vi "Pre Launch Init.vi"(11 "Nested in":refnum<class "Save tdms.lvclass">) -> (0 "error out":errorcluster, 3 "Nested out":refnum<class "Save tdms.lvclass">)   [LabVIEW 2019, in "Save tdms.lvlib" / "Save tdms.lvclass"]
doc: "(<B>Filename</B>: Actor Framework.lvlib:Actor.lvclass:Pre Launch Init.vi)\n\nDefines behavior that occurs after the Launch Nested Actor method is invoked but before the actor's Actor Core method begins running.\n\nBy default, this method does nothing. A descendant class may override it to define behavior."
uses:
  Save tdms.lvclass
  <vilib>/ActorFramework/Actor/Actor.lvclass
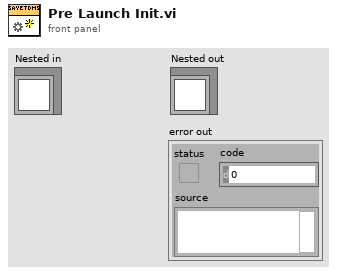
[diagram p1: front panel]
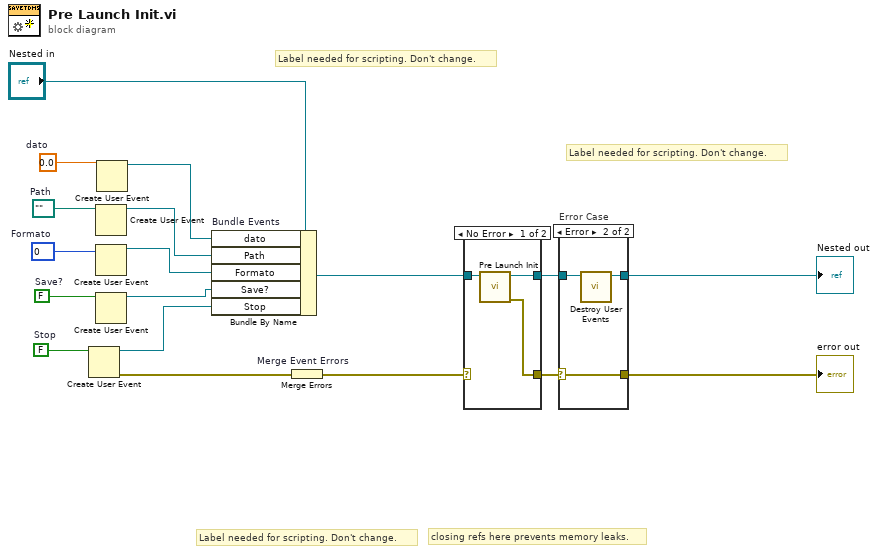
[diagram p0: block diagram]
diagram:
  w5 = 0.0  # dato
  w6 = path ""  # Path
  w7 = u16 0 items=[""]  # Formato
  w8 = FALSE  # Save?
  w17 = FALSE  # Stop
  # "Label needed for scripting. Don't change."
  # "Label needed for scripting. Don't change."
  # "Label needed for scripting. Don't change."
  # "closing refs here prevents memory leaks."
  n1 = Create User Event(user event datatype=w17) -> (user event=w14:refnum<user-event>, error out=w16:errorcluster)  [unwired: 1 in]
  n2 = Create User Event(user event datatype=w6) -> (user event=w3:refnum<user-event>)  [unwired: 1 in, 1 out]
  n3 = Create User Event(user event datatype=w7) -> (user event=w2:refnum<user-event>)  [unwired: 1 in, 1 out]
  n4 = Create User Event(user event datatype=w8) -> (user event=w1:refnum<user-event>)  [unwired: 1 in, 1 out]
  n5 = Create User Event(user event datatype=w5) -> (user event=w4:refnum<user-event>)  [unwired: 1 in, 1 out]
  n6 = Bundle By Name "Bundle Events"(cluster="Nested in", "dato"=w4, "Path"=w3, "Formato"=w2, "Save?"=w1, "Stop"=w14) -> (w11:refnum<class "Save tdms.lvclass">)
  n7 = Merge Errors "Merge Event Errors"(w16) -> (w10:errorcluster)
  n8 = case shown="No Error" w10 {
    selector: w10 -> [_ w23]
    tunnel: [w21 w22] -> w12
    tunnel: w11 -> [w20 w22]
    tunnel: [w19 w23] -> w9
    frame No Error {
      n9 = call-parent "Pre Launch Init.vi"("Actor in"=w20) -> ("error out"=w19:errorcluster, "Actor out"=w21:refnum<class "Save tdms.lvclass">)  [unwired: 9 in]
    }
    frame Error {
    }
  }
  n10 = case "Error Case" shown="Error" w9 {
    selector: w9 -> [w24 w28]
    tunnel: w12 -> [w25 w27]
    tunnel: [w25 w26] -> w15
    tunnel: [w24 w28] -> w13
    frame No Error {
    }
    frame Error {
      n11 = call "Destroy User Events.vi"("UI Template in"=w27) -> ("UI Template out"=w26:refnum<class "Save tdms.lvclass">)  [unwired: 10 in]
    }
  }
  "error out" <- w13
  "Nested out" <- w15
